vi "PlotButtonsResize.vi"(8 "error in (no error)":errorcluster, 9 "Plot Area:Position":T1, 10 "ShowPlotToolBar":refnum<vi>, 11 "PlotToolBar":refnum<vi>) -> (0 "error out":errorcluster)   [LabVIEW 2021, in "RocketPlot.lvlib"]
uses:
  RocketPlot.lvlib
  <vilib>/Utility/miscctls.llb/LVPositionTypeDef.ctl
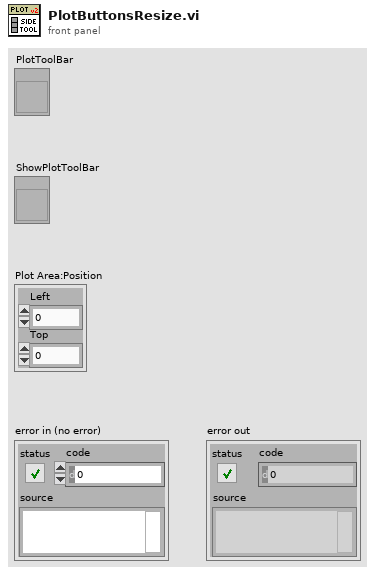
[diagram p1: front panel]
types:
  T1 = typedef "LVPositionTypeDef.ctl" = cluster{"Left":i32, "Top":i32}
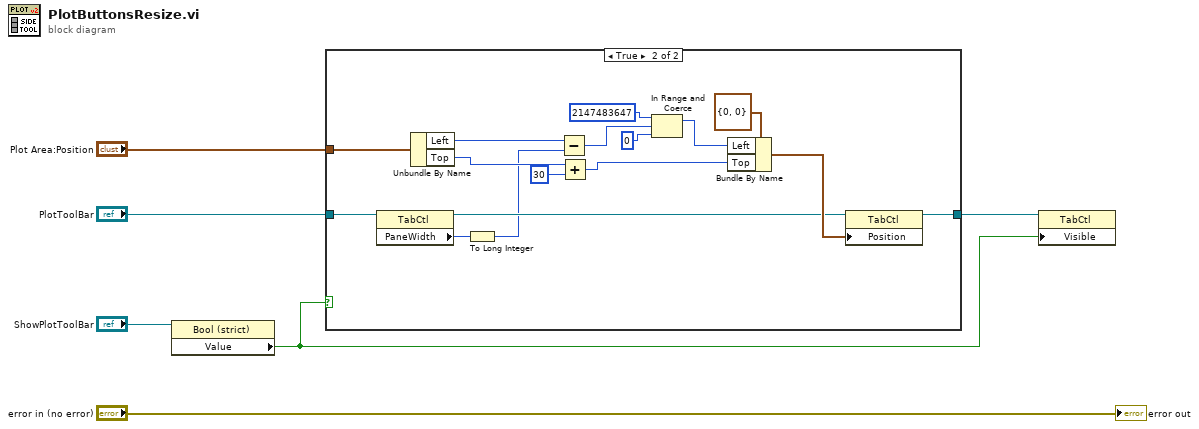
[diagram p0: block diagram]
diagram:
  n1 = property class="Bool (strict)"(reference="ShowPlotToolBar") -> ("Value"=w5:bool)  [unwired: 1 in, 2 out]
  n2 = case shown="True" w5 {
    tunnel: [w7 w23] -> w6
    tunnel: "PlotToolBar" -> [w7 w17]
    tunnel: "Plot Area:Position" -> [_ w16]
    frame False {
    }
    frame True {
      n3 = property class="TabCtl"(reference=w17) -> (reference out=w14:refnum<vi>, "PaneWidth"=w10:u32)  [unwired: 1 in, 1 out]
      n4 = Unbundle By Name(w16) -> ("Left"=w20:i32, "Top"=w21:i32)
      n5 = To Long Integer(number=w10) -> (32bit integer=w9:i32)
      n6 = Subtract(x=w20, y=w9) -> (x-y=w13:i32)
      n7 = Add(x=w21, y=30) -> (x+y=w22:i32)
      n8 = In Range and Coerce(upper limit=2147483647 ("lower limit"), x=w13, lower limit=0) -> (coerced(x)=w11:i32)  [unwired: 1 out]
      n9 = Bundle By Name(cluster=T1 {"Left"=0, "Top"=0} ("Position"), "Left"=w11, "Top"=w22) -> (w15:T1)
      n10 = property class="TabCtl"(reference=w14, "Position"=w15) -> (reference out=w23:refnum<vi>)  [unwired: 1 in, 1 out]
    }
  }
  n11 = property class="TabCtl"(reference=w6, "Visible"=w5) -> ()  [unwired: 1 in, 2 out]
  "error out" <- "error in (no error)"
